vi "DAQ.vi"(8 "error in (no error)":errorcluster, 10 "b":dbl=-4.09, 11 "m":dbl=2.35) -> (0 "error out":errorcluster, 1 "Force":dbl[](array[numeric]), 2 "Waveform Graph - Dark":dbl[](graph), 3 "Torque Array":dbl[](array[numeric]))   [LabVIEW 2020]
doc: "This VI adquires a voltage signal from a torque sensor/cell using the AI0 with a sample rate of 1000 Samples per second"
uses:
  <vilib>/numeric/Random Number (Range) DBL.vi
  <vilib>/DAQmx/read.llb/DAQmx Read (Analog DBL 1Chan 1Samp).vi
  <vilib>/DAQmx/create/channels.llb/DAQmx Create Channel (AI-Voltage-Basic).vi
  Global Variables/StopReadinf.vi
  <vilib>/DAQmx/configure/timing.llb/DAQmx Timing (Sample Clock).vi
  <vilib>/DAQmx/miscellaneous.llb/DAQmx Fill In Error Info.vi
  <vilib>/Analysis/NI_AALBase.lvlib
panel:
  out "Waveform Graph - Dark 2":dbl[](graph)
  in  "Distance":dbl=3.45
  out "Torque":dbl(graph) caption="Waveform Chart - Dark"
  out "Waveform Chart - Dark 2":dbl(graph) caption="Waveform Chart - Dark"
  in  "Cancel Button":bool
  out "Waveform Chart - Dark":dbl(graph)
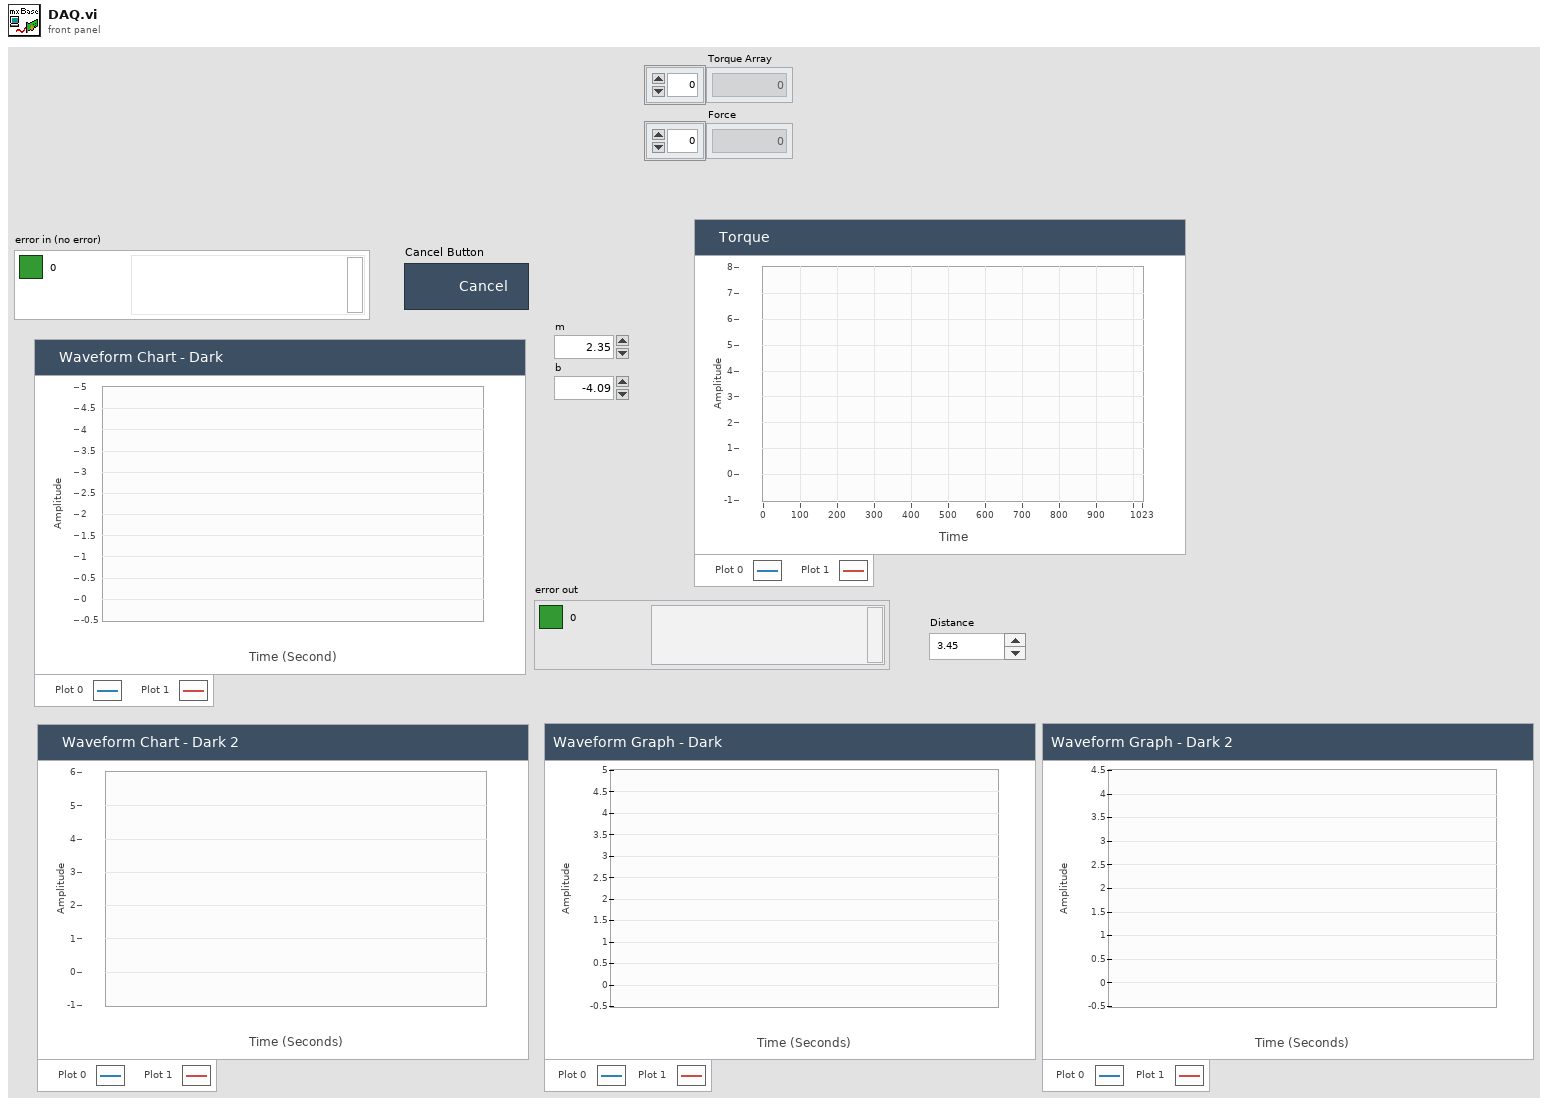
[diagram p1: front panel]
types:
  T1 = enum16{"Create Task", "Sampling Rate", "Start Reading", "Stop/Clear"}
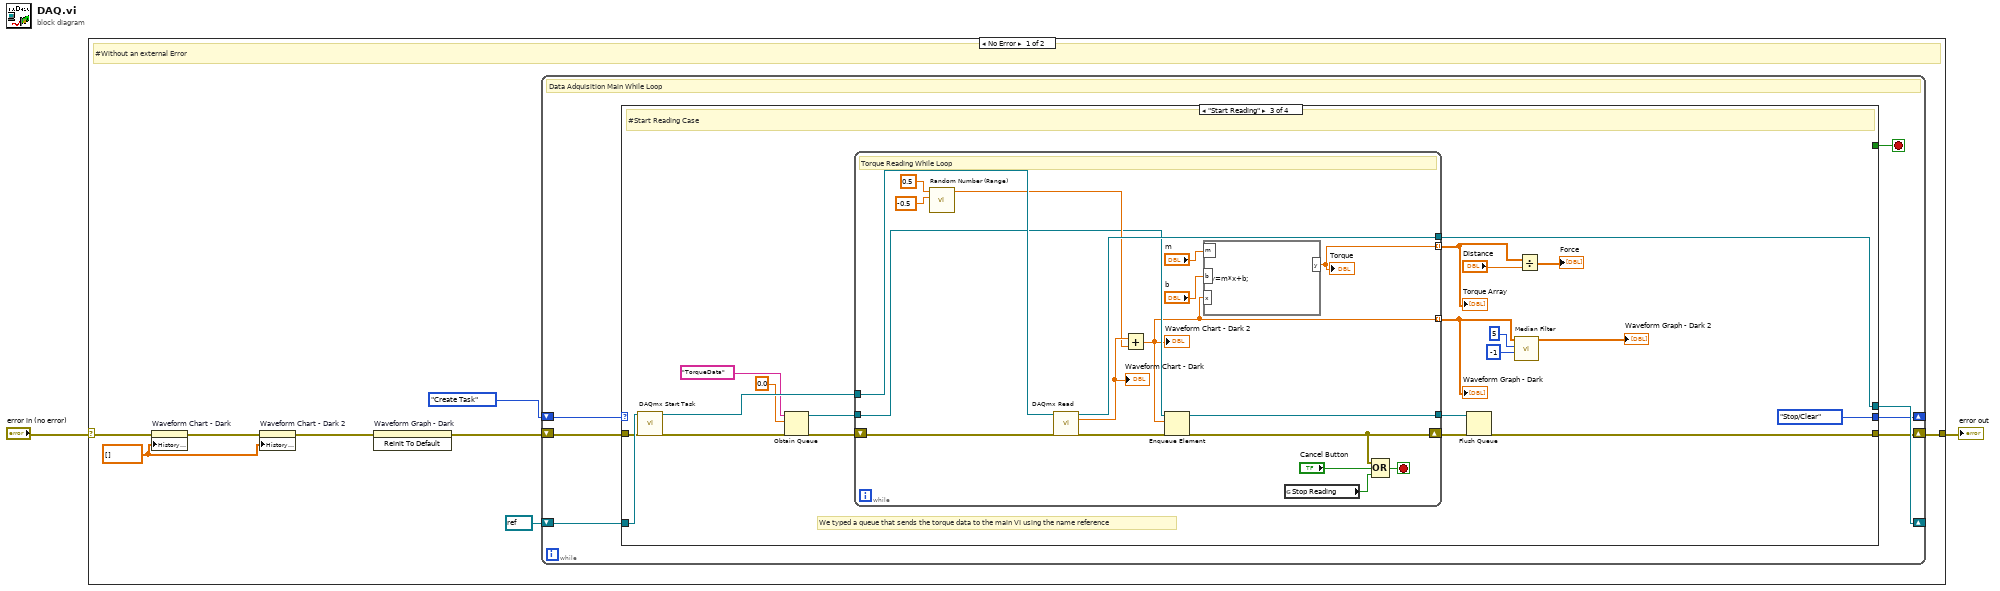
[diagram p0: block diagram]
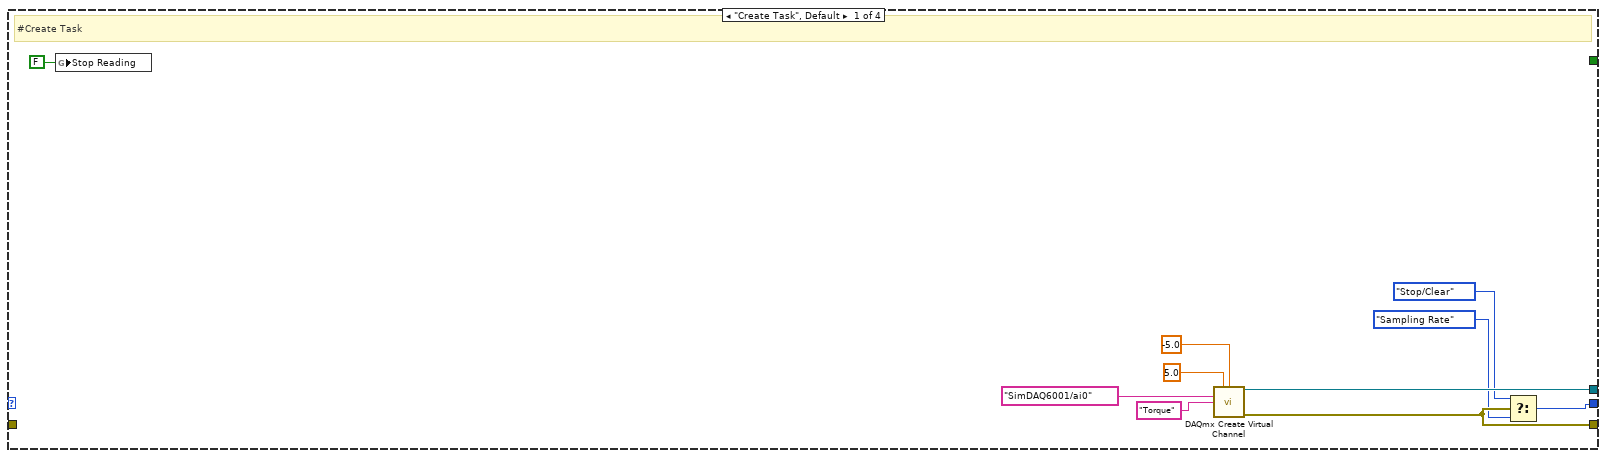
[diagram p2: hidden frame]
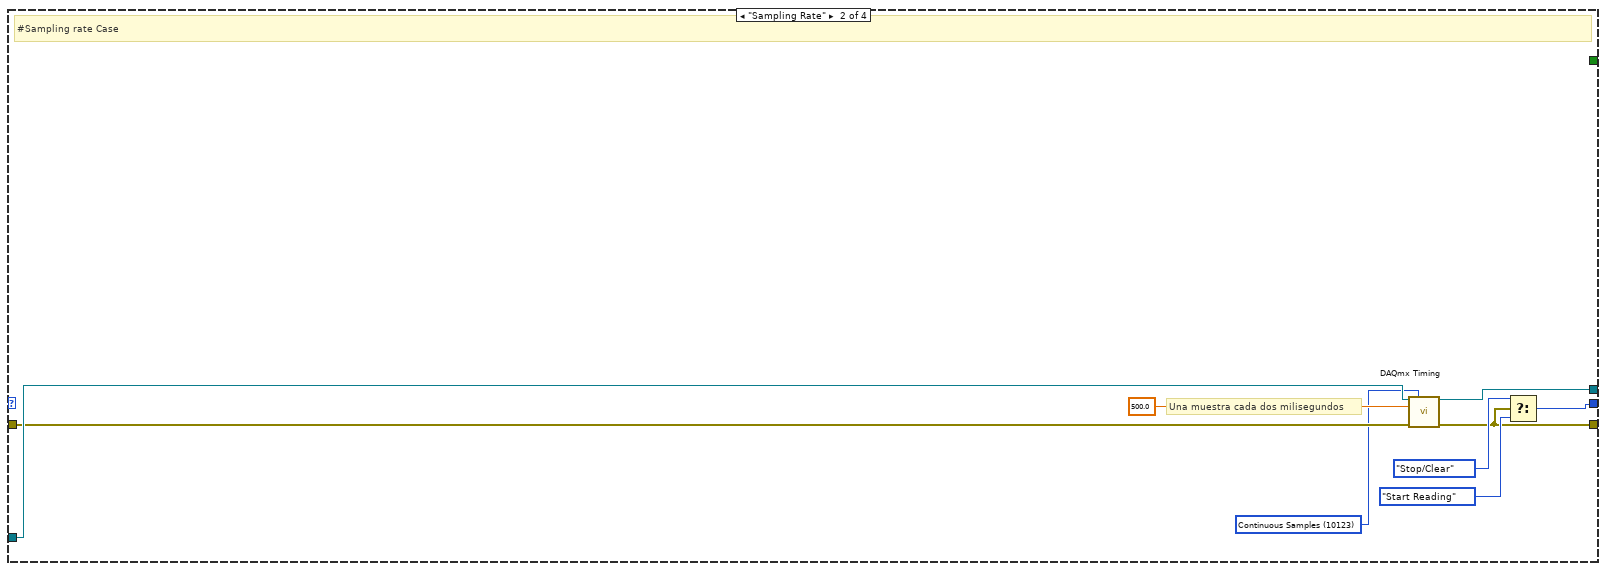
[diagram p3: hidden frame]
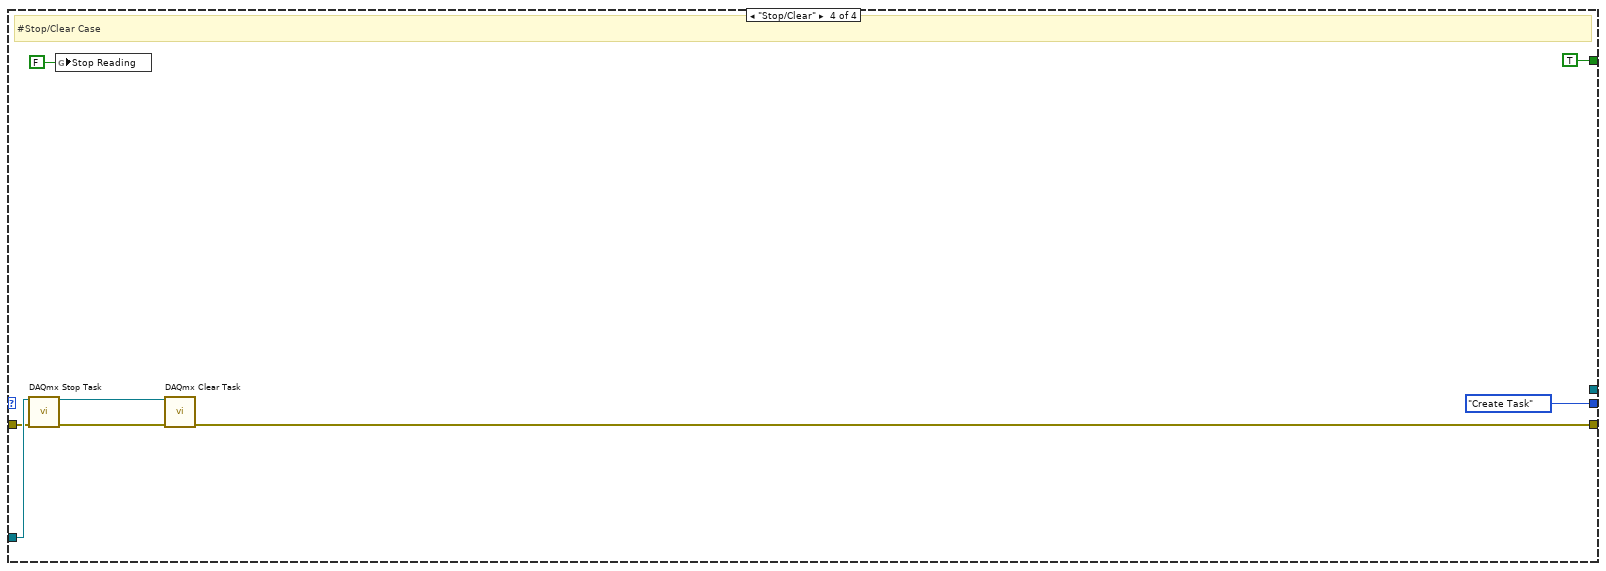
[diagram p4: hidden frame]
diagram:
  n1 = case shown="No Error" "error in (no error)" {
    selector: "error in (no error)" -> [w6 w83]
    tunnel: [w9 w83] -> w1
    frame No Error {
      w7 = dbl[] [] ("History Data")
      # "#Without an external Error"
      n2 = property on="Waveform Chart - Dark" class="WFChart (strict)"(error in=w6, "History Data"=w7) -> (error out=w5:errorcluster)  [unwired: 1 in, 1 out]
      n3 = property on="Waveform Chart - Dark 2" class="WFChart (strict)"(error in=w5, "History Data"=w7) -> (error out=w4:errorcluster)  [unwired: 1 in, 1 out]
      n4 = invoke on="Waveform Graph - Dark" class="WFGraph (strict)" method="Reinit To Default"(error in=w4) -> (error out=w3:errorcluster)  [unwired: 2 in, 2 out]
      n5 = while {
        shift-right: [w14] -> _
        shift-left: T1."Create Task" -> [w17]
        shift-right: [w16] -> _
        shift-left: refnum<k21> refnum ("task out") -> [w13]
        shift-right: [w15] -> w9
        shift-left: w3 -> [w12]
        stop <- w11 stop-if-true
        # "Data Adquisition Main While Loop"
        n6 = case shown="\"Start Reading\"" w17 {
          tunnel: [w25 w32 w53 _] -> w16
          tunnel: [w24 w29 w44 w78] -> w15
          tunnel: [w21 w28 T1."Stop/Clear" T1."Create Task"] -> w14
          tunnel: w13 -> [_ w36 w56 w82]
          tunnel: w12 -> [_ w35 w55 w81]
          tunnel: [_ _ _ TRUE] -> w11
          frame "Create Task", Default {
            # "#Create Task"
            n7 = global write "StopReadinf.vi" "Stop Reading"(FALSE ("Stop Reading")) -> ()
            n8 = call-poly <vilib>:"DAQmx Create Virtual Channel.vi"("maximum value"=5.0, "minimum value"=-5.0, "physical channels"=tag "SimDAQ6001/ai0", "name to assign"="Torque") -> ("task out"=w25:refnum<k21>, "error out"=w24:errorcluster)  [unwired: 10 in]
            n9 = Select(t=T1."Stop/Clear", s=w24, f=T1."Sampling Rate") -> (s? t:f=w21:T1)
          }
          frame "Sampling Rate" {
            w33 = 10123 items=["Finite Samples"=10178, "Continuous Samples"=10123, "Hardware Timed Single Point"=12522] ("sample mode")
            # "Una muestra cada dos milisegundos"
            # "#Sampling rate Case"
            n10 = call-poly <vilib>:"DAQmx Timing.vi"("task/channels in"=w36, "sample mode"=w33, "rate"=500.0, "error in"=w35) -> ("task out"=w32:refnum<k21>, "error out"=w29:errorcluster)  [unwired: 10 in]
            n11 = Select(t=T1."Stop/Clear", s=w29, f=T1."Start Reading") -> (s? t:f=w28:T1)
          }
          frame "Start Reading" {
            # "We typed a queue that sends the torque data to the main VI using the name reference"
            # "#Start Reading Case"
            n12 = call <vilib>:"DAQmx Start Task.vi"("task/channels in"=w56, "error in"=w55) -> ("task out"=w54:refnum<k21>, "error out"=w48:errorcluster)  [unwired: 12 in]
            n13 = Obtain Queue(name (unnamed)="TorqueData", element data type=0.0, error in (no error)=w48) -> (queue out=w49:refnum<queue>, error out=w47:errorcluster)  [unwired: 2 in, 1 out]
            n14 = while {
              tunnel: w54 -> [w74]
              tunnel: [w70] -> w53
              shift-right: [w62] -> w45
              shift-left: w47 -> [w73]
              tunnel: [w58] -> w40 mode=indexing
              tunnel: w49 -> [w65]
              tunnel: [w61] -> w46
              tunnel: [w57] -> w43 mode=indexing
              stop <- w71 stop-if-true
              # "Torque Reading While Loop"
              n15 = call-poly <vilib>:"Random Number (Range).vi"("lower bound (0)"=-0.5, "upper bound (100)"=0.5) -> ("number"=w66:dbl)  [unwired: 9 in]
              n16 = call-poly <vilib>:"DAQmx Read.vi"("task/channels in"=w74, "error in"=w73) -> ("task out"=w70:refnum<k21>, "data"=w67:dbl, "error out"=w64:errorcluster)  [unwired: 11 in]
              "Waveform Chart - Dark" <- w67
              n17 = Add(x=w67, y=w66) -> (x+y=w58:dbl)
              "Waveform Chart - Dark 2" <- w58
              n18 = Enqueue Element(queue=w65, element=w58, error in (no error)=w64) -> (queue out=w61:refnum<queue>, error out=w62:errorcluster)  [unwired: 1 in, 1 out]
              n19 = formula code="y=m*x+b;"("m"="m", "b"="b", "x"=w58) -> ("y"=w57:dbl)
              "Torque" <- w57
              n20 = global read "StopReadinf.vi" "Stop Reading"() -> (w63:bool)
              n21 = Compound Arithmetic op=OR(w62, "Cancel Button", w63) -> (w71:bool)
            }
            "Waveform Graph - Dark" <- w40
            "Torque Array" <- w43
            n22 = Flush Queue(queue=w46, error in (no error)=w45) -> (error out=w44:errorcluster)  [unwired: 2 out]
            n23 = call <vilib>:"Median Filter.vi"("right rank"=-1, "left rank"=5, "X"=w40) -> ("Filtered X"=→"Waveform Graph - Dark 2":dbl[])  [unwired: 7 in, 1 out]
            n24 = Divide(x=w43, y="Distance") -> (x/y=→"Force":dbl[])
          }
          frame "Stop/Clear" {
            # "#Stop/Clear Case"
            n25 = call <vilib>:"DAQmx Stop Task.vi"("task/channels in"=w82, "error in"=w81) -> ("task out"=w80:refnum<k21>, "error out"=w79:errorcluster)  [unwired: 12 in]
            n26 = global write "StopReadinf.vi" "Stop Reading"(FALSE ("Stop Reading")) -> ()
            n27 = call <vilib>:"DAQmx Clear Task.vi"("task in"=w80, "error in"=w79) -> ("error out"=w78:errorcluster)  [unwired: 13 in]
          }
        }
      }
    }
    frame Error {
      # "#With an external error"
    }
  }
  "error out" <- w1
